vi "Preloaded Comment.vi"(7 "QRD":T1, 8 "error in":errorcluster) -> (0 "error out":errorcluster, 5 "QRD Out":T1)   [LabVIEW 2025]
uses:
  Controls/Queues-Refs-Data.ctl
  Builds/Queue Wrappers.lvlibp/Q Packet.ctl
  Builds/Queue Wrappers.lvlibp
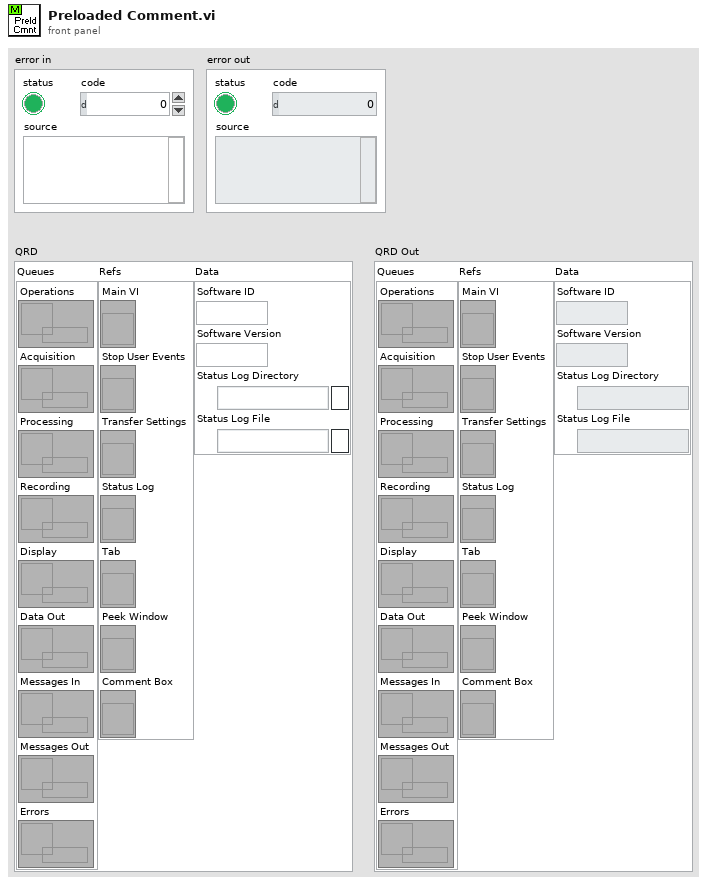
[diagram p1: front panel]
types:
  T1 = typedef "Queues-Refs-Data.ctl" = cluster{"Queues":cluster{"Operations":refnum<queue>, "Acquisition":refnum<queue>, "Processing":refnum<queue>, "Recording":refnum<queue>, "Display":refnum<queue>, "Data Out":refnum<queue>, "Messages In":refnum<queue>, "Messages Out":refnum<queue>, "Errors":refnum<queue>}, "Refs":cluster{"Main VI":refnum<vi>, "Stop User Events":refnum<vi>, "Transfer Settings":refnum<vi>, "Status Log":refnum<vi>, "Tab":refnum<vi>, "Peek Window":refnum<vi>, "Comment Box":refnum<vi>}, "Data":cluster{"Software ID":string, "Software Version":string, "Status Log Directory":path, "Status Log File":path}}
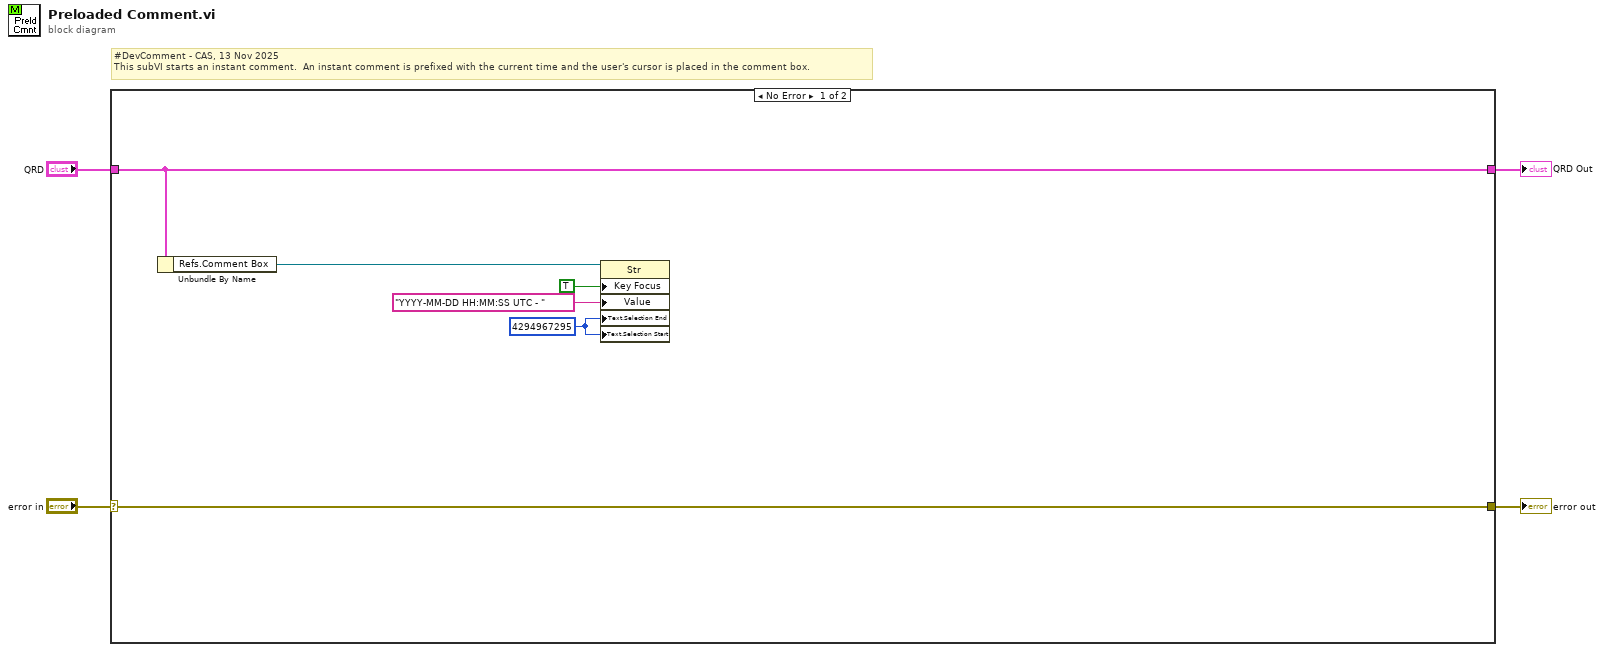
[diagram p0: block diagram]
diagram:
  # "#DevComment - CAS, 13 Nov 2025\nThis subVI starts an instant comment.  An instant comment is prefixed with the current time and the user's cursor is placed in the comment box."
  n1 = case shown="No Error" "error in" {
    selector: "error in" -> [w9 w12]
    tunnel: "QRD" -> [w7 w11]
    tunnel: [w9 w12] -> w2
    tunnel: [w7 w11] -> w1
    frame No Error {
      w5 = u32 4294967295 ("Text.Selection:End")
      n2 = Unbundle By Name(w7) -> ("Refs.Comment Box"=w10:refnum<vi>)
      n3 = property class="Str"(reference=w10, "Key Focus"=TRUE, "Value"="YYYY-MM-DD HH:MM:SS UTC - " ("time format string (%c)"), "Text.Selection End"=w5, "Text.Selection Start"=w5) -> ()  [unwired: 1 in, 2 out]
    }
    frame Error {
    }
  }
  "error out" <- w2
  "QRD Out" <- w1
